vi "DE_Initialize Parameter.vi"(10 "max bound":dbl, 11 "min bound":dbl) -> (3 "parameter":dbl)   [LabVIEW 2020, in "NI_AAL_GlobalOptimization.lvlib"]
uses:
  <vilib>/gmath/NI_AAL_GlobalOptimization.lvlib
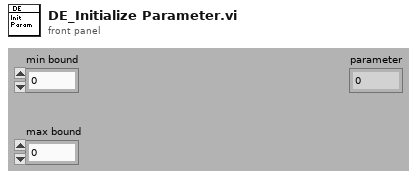
[diagram p1: front panel]
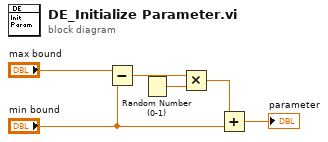
[diagram p0: block diagram]
diagram:
  n1 = Subtract(x="max bound", y="min bound") -> (x-y=w3:dbl)
  n2 = Random Number (0-1)() -> (number: 0 to 1=w1:dbl)
  n3 = Multiply(x=w3, y=w1) -> (x*y=w2:dbl)
  n4 = Add(x=w2, y="min bound") -> (x+y=→"parameter":dbl)
